vi "ReadAllCtlRefs.vi"(8 "error in (no error)":errorcluster, 11 "CtlLookup In":T1) -> (0 "error out":errorcluster, 1 "CtlRef Array":refnum<vi>[](array[refnum]), 2 "CtlName Array":string[](array[string]), 3 "CtlLookup Out":T1)   [LabVIEW 2020, in "CtlReferences.lvlib" / "CtlReferences.lvclass"]
doc: "Read all Refs from DVR"
uses:
  CtlReferences.lvclass
  TypeDefs/CtlLookup.ctl
  CtlReferences.lvclass/CtlReferences.ctl
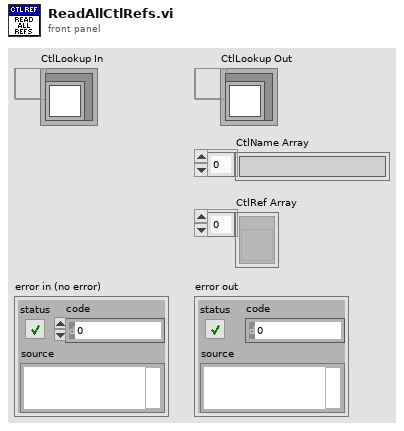
[diagram p1: front panel]
types:
  T1 = typedef "CtlReferences.lvlib/CtlReferences.lvclass/CtlLookup.ctl" = refnum<data-value>
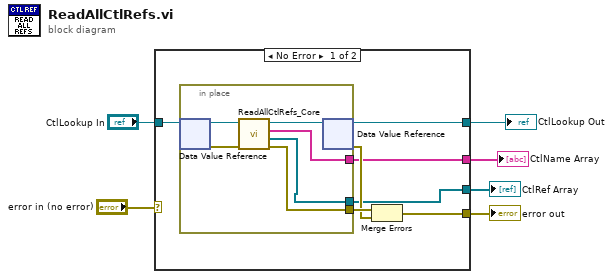
[diagram p0: block diagram]
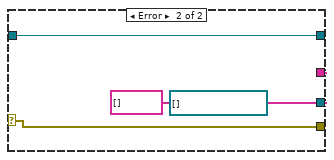
[diagram p2: hidden frame]
diagram:
  n1 = case shown="No Error" "error in (no error)" {
    selector: "error in (no error)" -> [_ w23]
    tunnel: "CtlLookup In" -> [w13 w21]
    tunnel: [w7 w23] -> w1
    tunnel: [w10 string[] []] -> w4
    tunnel: [w9 w21] -> w6
    tunnel: [w8 refnum<vi>[] []] -> w2
    frame No Error {
      n2 = in-place {
        in-place-border: [w18] -> w10
        in-place-border: [w17] -> w8
        in-place-border: [w16] -> w12
        n3 = in-place-dvr #1(w13) -> (w15:refnum<class "CtlReferences.lvclass">, w19:errorcluster)
        n4 = call-dynamic "ReadAllCtlRefs_Core.vi"("error in (no error)"=w19, "CtlReferences in"=w15) -> ("error out"=w16:errorcluster, "Values"=w17:refnum<vi>[], "Names"=w18:string[], "CtlReferences out"=w14:refnum<class "CtlReferences.lvclass">)  [unwired: 6 in]
        n5 = in-place-dvr #1(w14) -> (w9:T1, w11:errorcluster)
      }
      n6 = Merge Errors(w12, w11) -> (w7:errorcluster)
    }
    frame Error {
    }
  }
  "CtlLookup Out" <- w6
  "CtlName Array" <- w4
  "error out" <- w1
  "CtlRef Array" <- w2
